vi "start_data_file.vi"(6 "gas flow rate":string, 7 "DataFile":path, 8 "sample volume":string, 9 "sample type":string, 10 "iteration":dbl, 11 "sample id":string) -> (0 "error out":errorcluster, 3 "Byte Stream File Refnum":refnum<file>)   [LabVIEW 2010]
panel:
  # "integral from LiCor"
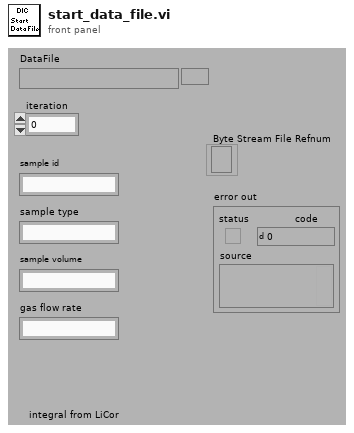
[diagram p1: front panel]
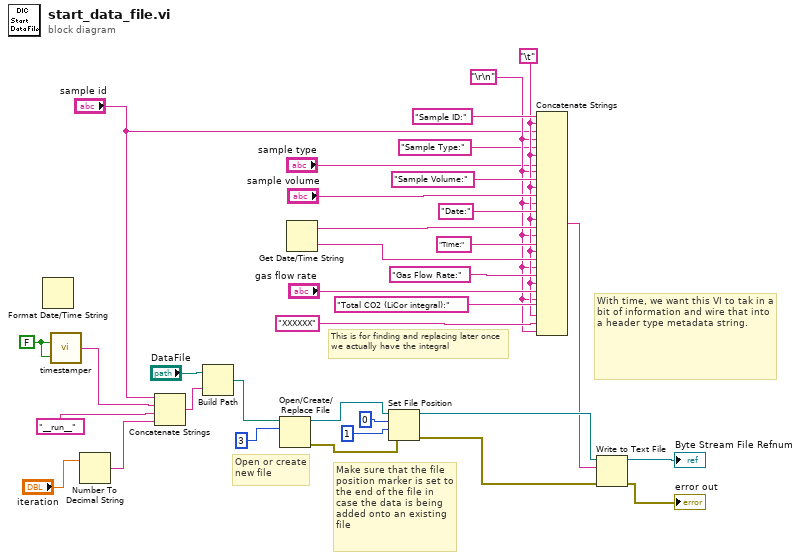
[diagram p0: block diagram]
diagram:
  w3 = FALSE
  w7 = "\t"
  w6 = "\r\n"
  # "This is for finding and replacing later once we actually have the integral"
  # "Make sure that the file position marker is set to the end of the file in case the data is being added onto an existing file"
  # "With time, we want this VI to tak in a bit of information and wire that into a header type metadata string."
  # "Open or create new file"
  n1 = Format Date/Time String() -> ()  [unwired: 3 in, 1 out]
  n2 = call "timestamper.vi"("seconds?"=w3, "ms?"=w3) -> ("datetime output"=w2:string)
  n3 = Number To Decimal String(number="iteration") -> (decimal integer string=w30:string)  [unwired: 1 in]
  n4 = Concatenate Strings("sample id", w2, "__run__", w30) -> (w29:string)
  n5 = Build Path(base path="DataFile", name or relative path=w29) -> (appended path=w28:path)
  n6 = Open/Create/Replace File(file path (use dialog)=w28, operation (0:open)=3) -> (refnum out=w21:refnum<file>, error out=w24:errorcluster)  [unwired: 4 in, 1 out]
  n7 = Get Date/Time String() -> (date string=w17:string, time string=w15:string)  [unwired: 3 in]
  n8 = Set File Position(offset (in bytes) (0)=0, refnum=w21, from (0:start)=1, error in=w24) -> (refnum out=w22:refnum<file>, error out=w23:errorcluster)
  n9 = Concatenate Strings("Sample ID:", w7, "sample id", w6, "Sample Type:", w7, "sample type", w6, "Sample Volume:", w7, "sample volume", w6, "Date:", w7, w17, w6, "Time:", w7, w15, w6, "Gas Flow Rate:", w7, "gas flow rate", w6, "Total CO2 (LiCor integral):", w7, "XXXXXX", w6) -> (w11:string)
  n10 = Write to Text File(file (use dialog)=w22, text=w11, error in=w23) -> (refnum out=→"Byte Stream File Refnum":refnum<file>, error out=→"error out":errorcluster)  [unwired: 1 in, 1 out]
